vi "Update Normalized Axes.vi"(8 "axis in":T2, 11 "Device in":T1={"device ID"=refnum, "Device Name"="Logitech Extreme 3D", "axis info"={"X axis"=[], "Y axis"=[], "Z axis"=[], "X axis rotation"=[], "Y axis rotation"=[], "Z axis rotation"=[], "U axis"=[], "V axis"=[]}}) -> (0 "axis out":T2, 3 "Device out":T1={"device ID"=refnum, "Device Name"="Logitech Extreme 3D", "axis info"={"X axis"=[], "Y axis"=[], "Z axis"=[], "X axis rotation"=[], "Y axis rotation"=[], "Z axis rotation"=[], "U axis"=[], "V axis"=[]}})   [LabVIEW 2012]
doc: "This VI simply contains the mathematical logic necessary to discern a new global maximum or minimum for each unique axis available.\nRuffin"
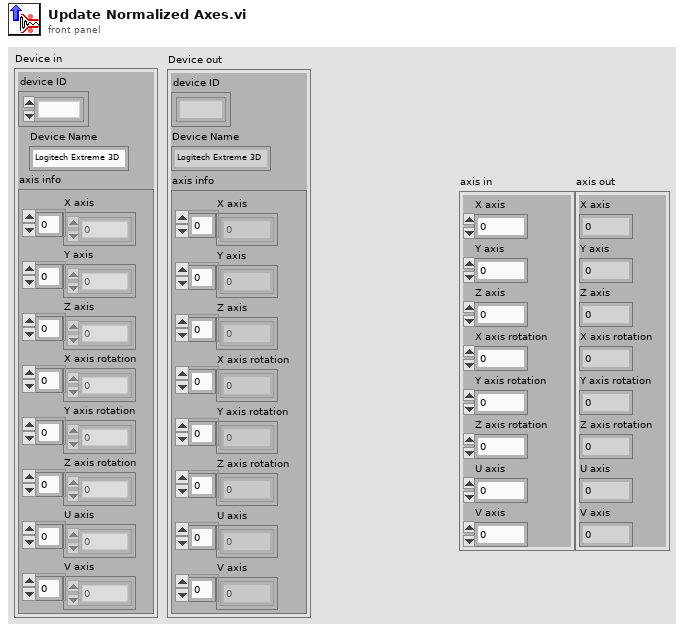
[diagram p1: front panel]
types:
  T1 = cluster{"device ID":refnum<k1>, "Device Name":string, "axis info":cluster{"X axis":dbl[], "Y axis":dbl[], "Z axis":dbl[], "X axis rotation":dbl[], "Y axis rotation":dbl[], "Z axis rotation":dbl[], "U axis":dbl[], "V axis":dbl[]}}
  T2 = cluster{"X axis":i32, "Y axis":i32, "Z axis":i32, "X axis rotation":i32, "Y axis rotation":i32, "Z axis rotation":i32, "U axis":i32, "V axis":i32}
  T3 = cluster{"X axis":dbl[], "Y axis":dbl[], "Z axis":dbl[], "X axis rotation":dbl[], "Y axis rotation":dbl[], "Z axis rotation":dbl[], "U axis":dbl[], "V axis":dbl[]}
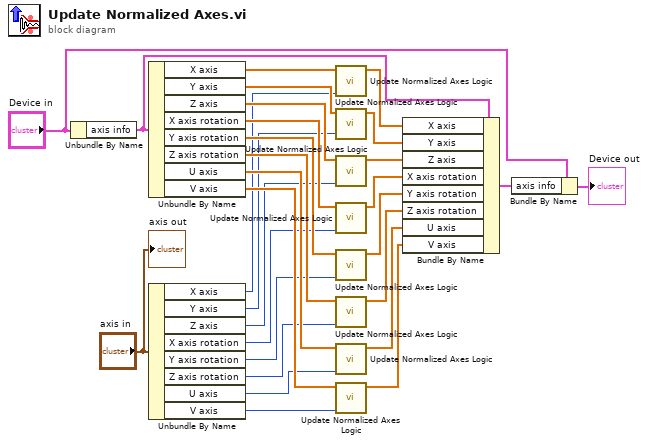
[diagram p0: block diagram]
diagram:
  n1 = Unbundle By Name("Device in") -> ("axis info"=w25:T3)
  n2 = Unbundle By Name(w25) -> ("X axis"=w24:dbl[], "Y axis"=w22:dbl[], "Z axis"=w21:dbl[], "X axis rotation"=w20:dbl[], "Y axis rotation"=w19:dbl[], "Z axis rotation"=w18:dbl[], "U axis"=w17:dbl[], "V axis"=w16:dbl[])
  n3 = Unbundle By Name("axis in") -> ("X axis"=w15:i32, "Y axis"=w14:i32, "Z axis"=w13:i32, "X axis rotation"=w12:i32, "Y axis rotation"=w11:i32, "Z axis rotation"=w10:i32, "U axis"=w9:i32, "V axis"=w8:i32)
  n4 = call "Update Normalized Axes Logic.vi"("axis"=w15, "axis in"=w24) -> ("axis out"=w23:dbl[])  [unwired: 9 in]
  n5 = call "Update Normalized Axes Logic.vi"("axis"=w14, "axis in"=w22) -> ("axis out"=w1:dbl[])  [unwired: 9 in]
  n6 = call "Update Normalized Axes Logic.vi"("axis"=w13, "axis in"=w21) -> ("axis out"=w2:dbl[])  [unwired: 9 in]
  n7 = call "Update Normalized Axes Logic.vi"("axis"=w12, "axis in"=w20) -> ("axis out"=w3:dbl[])  [unwired: 9 in]
  n8 = call "Update Normalized Axes Logic.vi"("axis"=w11, "axis in"=w19) -> ("axis out"=w4:dbl[])  [unwired: 9 in]
  n9 = call "Update Normalized Axes Logic.vi"("axis"=w10, "axis in"=w18) -> ("axis out"=w5:dbl[])  [unwired: 9 in]
  n10 = call "Update Normalized Axes Logic.vi"("axis"=w9, "axis in"=w17) -> ("axis out"=w6:dbl[])  [unwired: 9 in]
  n11 = call "Update Normalized Axes Logic.vi"("axis"=w8, "axis in"=w16) -> ("axis out"=w7:dbl[])  [unwired: 9 in]
  n12 = Bundle By Name(cluster=w25, "X axis"=w23, "Y axis"=w1, "Z axis"=w2, "X axis rotation"=w3, "Y axis rotation"=w4, "Z axis rotation"=w5, "U axis"=w6, "V axis"=w7) -> (w26:T3)
  n13 = Bundle By Name(cluster="Device in", "axis info"=w26) -> (→"Device out":T1)
  "axis out" <- "axis in"
